vi "Set.vi"(8 "error in (no error)":errorcluster, 9 "Acceleration":dbl, 10 "Velocity":dbl, 11 "Queue Name":string) -> (0 "error out":errorcluster)   [LabVIEW 2019, in "ADLINK Motion Card.lvlib"]
uses:
  ADLINK Motion Card.lvlib
  Queues/Message Cluster.ctl
  SEQ/SEQ Data.ctl
  Queues/Queues.lvlib
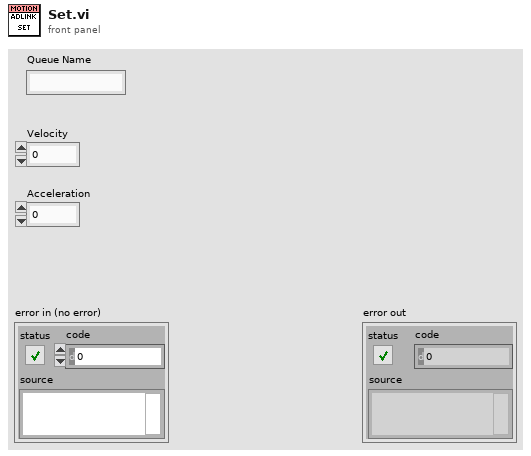
[diagram p1: front panel]
types:
  T1 = typedef "ADLINK Motion Card.lvlib/SEQ Data.ctl" = cluster{"Current Position":dbl, "Target Position":dbl, "Velocity":dbl, "Acceleration":dbl, "Arrived?":bool, "data value reference":refnum<data-value>, "VI Refnum":refnum<vi>}
  T2 = typedef "Queues.lvlib/Message Cluster.ctl" = cluster{"State":string, "Data":variant}
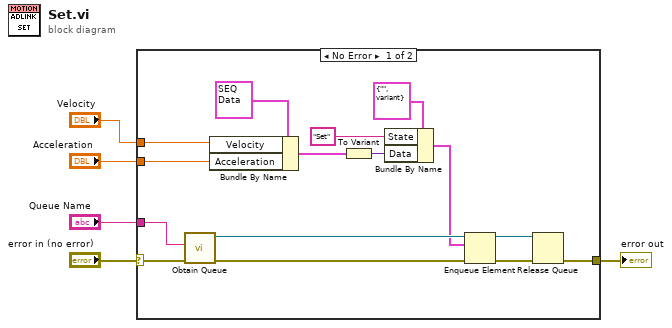
[diagram p0: block diagram]
diagram:
  n1 = case shown="No Error" "error in (no error)" {
    selector: "error in (no error)" -> [w19 w21]
    tunnel: "Queue Name" -> [w20 _]
    tunnel: [w12 w21] -> w3
    tunnel: "Velocity" -> [w7 _]
    tunnel: "Acceleration" -> [w6 _]
    frame No Error {
      n2 = call "Obtain Queue.vi"("Error In"=w19, "Queue Name"=w20) -> ("Error Out"=w18:errorcluster, "queue out"=w17:refnum<queue>)  [unwired: 8 in]
      n3 = Bundle By Name(cluster=T1 {"Current Position"=0.0, "Target Position"=0.0, "Velocity"=0.0, "Acceleration"=0.0, "Arrived?"=FALSE, "data value reference"=refnum, "VI Refnum"=refnum} ("SEQ Data"), "Velocity"=w7, "Acceleration"=w6) -> (w9:T1)
      n4 = To Variant(anything=w9) -> (Variant=w8:variant)
      n5 = Bundle By Name(cluster=T2 {"State"="", "Data"=variant} ("element"), "State"="Set", "Data"=w8) -> (w15:T2)
      n6 = Enqueue Element(queue=w17, element=w15, error in (no error)=w18) -> (queue out=w13:refnum<queue>, error out=w14:errorcluster)  [unwired: 1 in, 1 out]
      n7 = Release Queue(queue=w13, error in (no error)=w14) -> (error out=w12:errorcluster)  [unwired: 1 in, 2 out]
    }
    frame Error {
    }
  }
  "error out" <- w3
